vi "acc_gyro_logger.vi"() -> ()   [LabVIEW 2012]
uses:
  acc_gyro_data.ctl
  <vilib>/Instr/_visa.llb/VISA Configure Serial Port (Instr).vi
panel:
  out "Rate":dbl[unit]
  in  "Baud rate":u32=57600
  out "Accelerometer":waveform(dbl)[](graph)
  out "Gyro":waveform(dbl)[](graph)
  in  "accel range (m/s2)":dbl(ring)=8.0 items=["2"=2.0, "4"=4.0, "8"=8.0, "16"=16.0]
  in  "gyro range (deg/s)":dbl(ring)=250.0 items=["250"=250.0, "500"=500.0, "1000"=1000.0, "2000"=2000.0]
  in  "Serial port":refnum<visa-resource-name>="COM3"
  in  "stop":bool
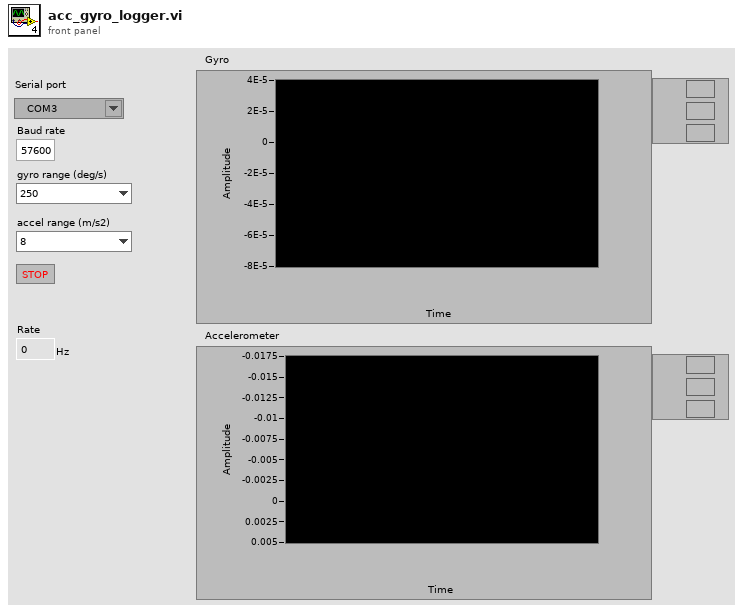
[diagram p1: front panel]
types:
  T1 = typedef "acc_gyro_data.ctl" = cluster{"milliseconds":u64, "gyro_x":dbl, "gyro_y":dbl, "gyro_z":dbl, "acc_x":dbl, "acc_y":dbl, "acc_z":dbl}
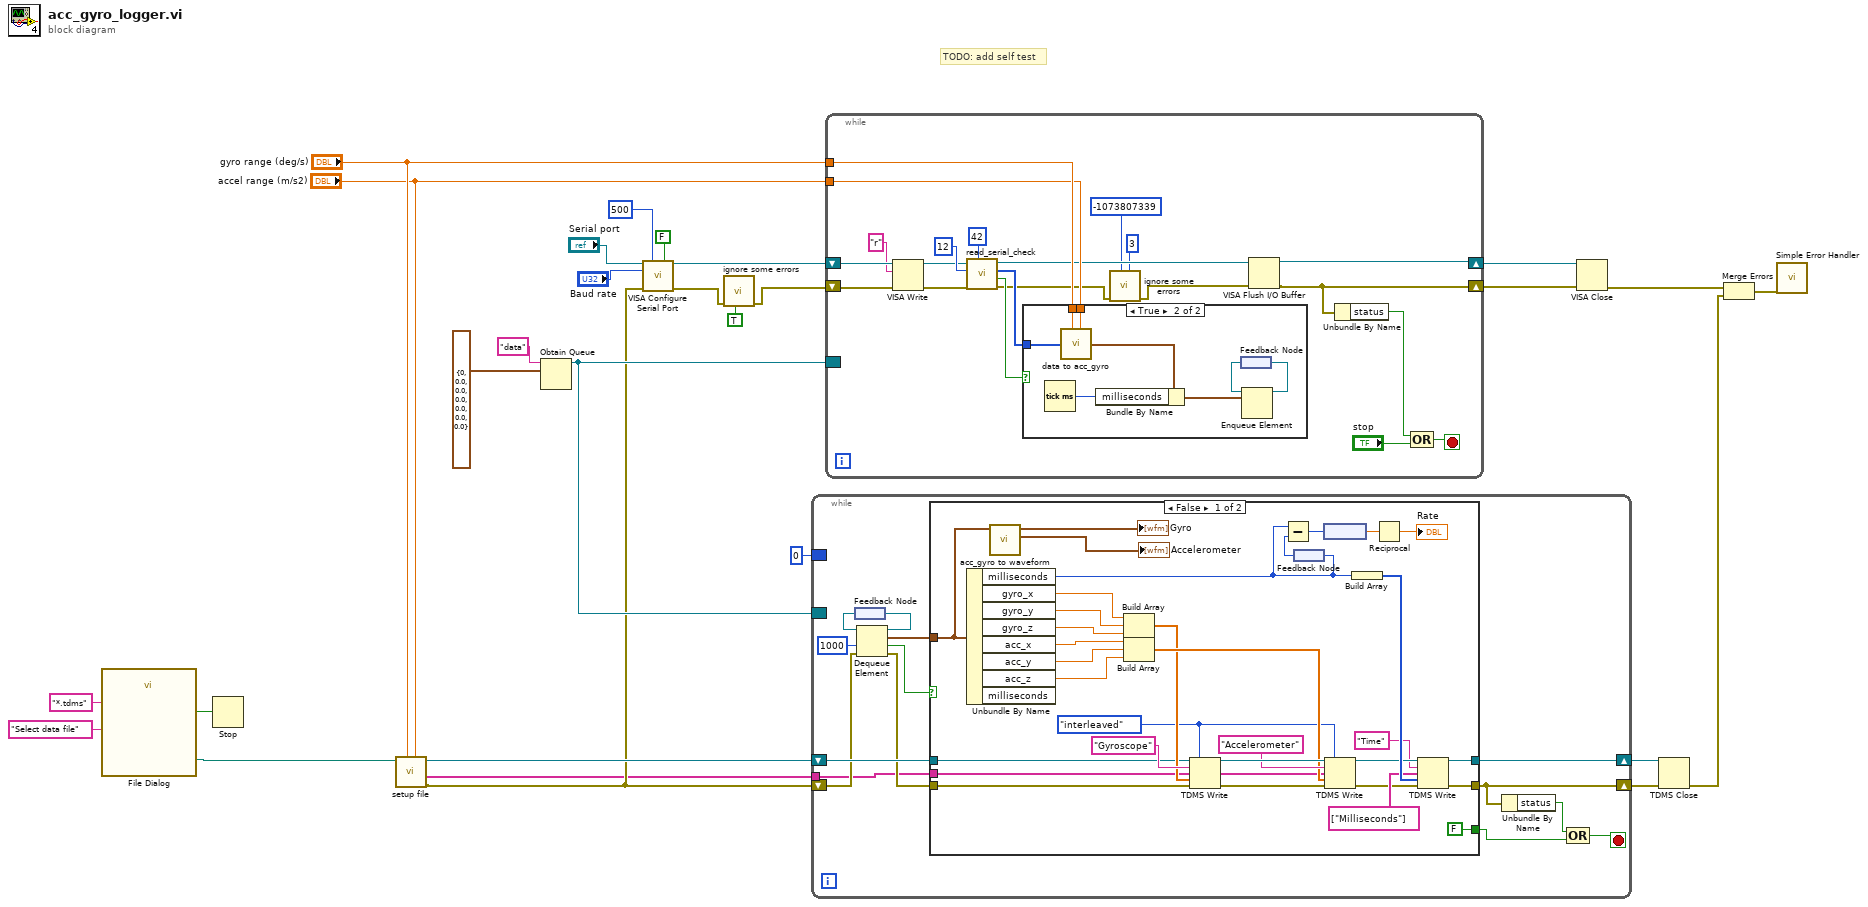
[diagram p0: block diagram]
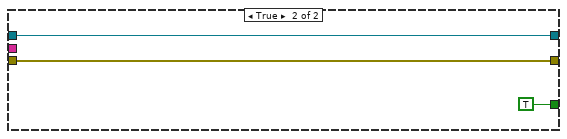
[diagram p2: hidden frame]
diagram:
  # "TODO: add self test"
  n1 = call "File Dialog"("prompt"="Select data file", "pattern (all files)"="*.tdms") -> ("selected path"=w21:path, "cancelled"=w20:bool)  [unwired: 10 in, 2 out]
  n2 = Stop(stop? (T)=w20) -> ()
  n3 = call "setup file.vi"("accel range"="accel range (m/s2)", "gyro range"="gyro range (deg/s)", "selected path"=w21) -> ("error out"=w10:errorcluster, "channel names"=w7:string[], "tdms file out"=w11:refnum<k34>)  [unwired: 6 in]
  n4 = Obtain Queue(name (unnamed)="data", element data type=T1 {"milliseconds"=0, "gyro_x"=0.0, "gyro_y"=0.0, "gyro_z"=0.0, "acc_x"=0.0, "acc_y"=0.0, "acc_z"=0.0} ("acc gyro data")) -> (queue out=w19:refnum<queue>)  [unwired: 3 in, 2 out]
  n5 = call-poly "VISA Configure Serial Port"("VISA resource name"="Serial port", "timeout (10sec)"=u32 500, "Enable Termination\nChar (T)"=FALSE ("Enable Termination\nChar (T)"), "baud rate (9600)"="Baud rate", "error in (no error)"=w10) -> ("VISA resource name out"=w4:refnum<visa-resource-name>, "error out"=w3:errorcluster)  [unwired: 9 in]
  n6 = call "ignore some errors.vi"("reset"=TRUE, "error in"=w3) -> ("error out"=w2:errorcluster)  [unwired: 9 in]
  n7 = while {
    border: w19 -> [_]
    shift-right: [w33] -> w16
    shift-left: w10 -> [w36]
    shift-right: [w38] -> w15
    shift-left: w11 -> [w39]
    tunnel: w7 -> [w29]
    border: u64 0 ("milliseconds") -> [_]
    stop <- w30 stop-if-true
    n8 = feedback #1() -> (w42:refnum<queue>)
    n9 = Dequeue Element(queue=w42, timeout in ms (-1)=1000, error in (no error)=w36) -> (queue out=w41:refnum<queue>, element=w40:T1, timed out?=w34:bool, error out=w35:errorcluster)
    n10 = feedback-in #1(w41) -> ()
    n11 = case shown="False" w34 {
      tunnel: w40 -> [w60 _]
      tunnel: [w51 w76] -> w33
      tunnel: w39 -> [w49 w77]
      tunnel: [w50 w77] -> w38
      tunnel: w35 -> [w52 w76]
      tunnel: [FALSE TRUE] -> w31
      tunnel: w29 -> [w57 _]
      frame False {
        w48 = enum16{"decimated", "interleaved"}."interleaved" ("data layout (0:decimated)")
        n12 = Unbundle By Name(w60) -> ("milliseconds"=w47:u64, "gyro_x"=w75:dbl, "gyro_y"=w74:dbl, "gyro_z"=w73:dbl, "acc_x"=w72:dbl, "acc_y"=w71:dbl, "acc_z"=w70:dbl)  [unwired: 1 out]
        n13 = call "acc_gyro to waveform.vi"("acc gyro data"=w60) -> ("accel plot"=→"Accelerometer":waveform(dbl)[], "gyro plot"=→"Gyro":waveform(dbl)[])  [unwired: 9 in]
        n14 = Build Array(w75, w74, w73) -> (w61:dbl[])
        n15 = Build Array(w72, w71, w70) -> (w65:dbl[])
        n16 = TDMS Write(0:w49, 1:w48, 5:"Gyroscope" ("group name (Untitled)"), 7:w57, 9:w61, 11:w52) -> (4:w68:refnum<k34>, 8:w56:string[], 15:w67:errorcluster)  [unwired: 1 out]
        n17 = feedback #2() -> (w46:u64)
        n18 = Subtract(x=w47, y=w46) -> (x-y=w45:u64)
        n19 = feedback-in #2(w47) -> ()
        n20 = node(w45) -> (w44:dbl[unit])
        n21 = TDMS Write(0:w68, 1:w48, 5:"Accelerometer" ("group name (Untitled)"), 7:w56, 9:w65, 11:w67) -> (4:w55:refnum<k34>, 15:w54:errorcluster)  [unwired: 2 out]
        n22 = Build Array(w47) -> (w64:u64[])
        n23 = Reciprocal(x=w44) -> (1/x=→"Rate":dbl[unit])
        n24 = TDMS Write(0:w55, 5:"Time" ("group name (Untitled)"), 7:string[] ["Milliseconds"] ("channel name(s) in (Untitled)"), 9:w64, 11:w54) -> (4:w50:refnum<k34>, 15:w51:errorcluster)  [unwired: 1 in, 2 out]
      }
      frame True {
      }
    }
    n25 = Unbundle By Name(w33) -> ("status"=w32:bool)
    n26 = Compound Arithmetic op=OR(w32, w31) -> (w30:bool)
  }
  n27 = while {
    tunnel: "gyro range (deg/s)" -> [w94]
    tunnel: "accel range (m/s2)" -> [w93]
    border: w19 -> [_]
    shift-right: [w83] -> w18
    shift-left: w2 -> [w90]
    shift-right: [w84] -> w17
    shift-left: w4 -> [w99]
    stop <- w87 stop-if-true
    n28 = VISA Write(VISA resource name=w99, write buffer="r", error in (no error)=w90) -> (VISA resource name out=w92:refnum<visa-resource-name>, error out=w89:errorcluster)  [unwired: 1 out]
    n29 = call "read_serial_check.vi"("checkval"=u8 42, "error in (no error)"=w89, "byte count"=u32 12, "VISA resource name"=w92) -> ("error out"=w82:errorcluster, "good"=w96:bool, "data"=w95:u8[], "VISA resource out"=w85:refnum<visa-resource-name>)  [unwired: 4 in]
    n30 = case shown="True" w96 {
      tunnel: w95 -> [_ w107]
      tunnel: w94 -> [_ w106]
      tunnel: w93 -> [_ w105]
      frame False {
      }
      frame True {
        n31 = Tick Count (ms)() -> (millisecond timer value=w102:u32)
        n32 = call "data to acc_gyro.vi"("byte array"=w107, "gyro range (deg/s)"=w106, "accel range (m/s2)"=w105) -> ("acc gyro data"=w101:T1)
        n33 = Bundle By Name(cluster=w101, "milliseconds"=w102) -> (w100:T1)
        n34 = feedback #3() -> (w103:refnum<queue>)
        n35 = Enqueue Element(queue=w103, element=w100) -> (queue out=w104:refnum<queue>)  [unwired: 2 in, 2 out]
        n36 = feedback-in #3(w104) -> ()
      }
    }
    n37 = call "ignore some errors.vi"("max errors"=3, "error code"=-1073807339, "error in"=w82) -> ("error out"=w81:errorcluster)  [unwired: 8 in]
    n38 = VISA Flush I/O Buffer(VISA resource name=w85, error in (no error)=w81) -> (VISA resource name out=w84:refnum<visa-resource-name>, error out=w83:errorcluster)  [unwired: 1 in]
    n39 = Unbundle By Name(w83) -> ("status"=w86:bool)
    n40 = Compound Arithmetic op=OR(w86, "stop") -> (w87:bool)
  }
  n41 = VISA Close(VISA resource name=w17, error in (no error)=w18) -> (error out=w14:errorcluster)
  n42 = TDMS Close(8:w16, 11:w15) -> (0:w13:errorcluster)  [unwired: 1 out]
  n43 = Merge Errors(w14, w13) -> (w12:errorcluster)
  n44 = call <vilib>:"Simple Error Handler.vi"("error in (no error)"=w12) -> ()  [unwired: 4 in, 5 out]
